vi "projekt2.vi"() -> ()   [LabVIEW 2020]
uses:
  6dc693d6-3625-4d42-a112-a50989b43f3c.vi
panel:
  in  "Precyzja":sgl min=0 max=6 step=1 format="%#_1g"
  out "Wynikk":string
  in  "Tryb":bool
  out "Wyniki":dbl(graph)
  out "Nieprawid³owa \nkonwersja":bool
  in  "Skala temperatury":bool
  in  "?":bool
  in  "stop":bool
  in  "Model [0-1]":u8 max=1 step=1
  in  "Rezystancja [DBL]":dbl format="%#.6g"
  in  "Jednostka [0-2]":u8 max=2 step=1
  # "Rezystancja"
  # "Temperatura"
  # "Czujnik"
  # "PT100"
  # "KTY81-210"
  # "Celcjusza"
  # "Fahrenheita"
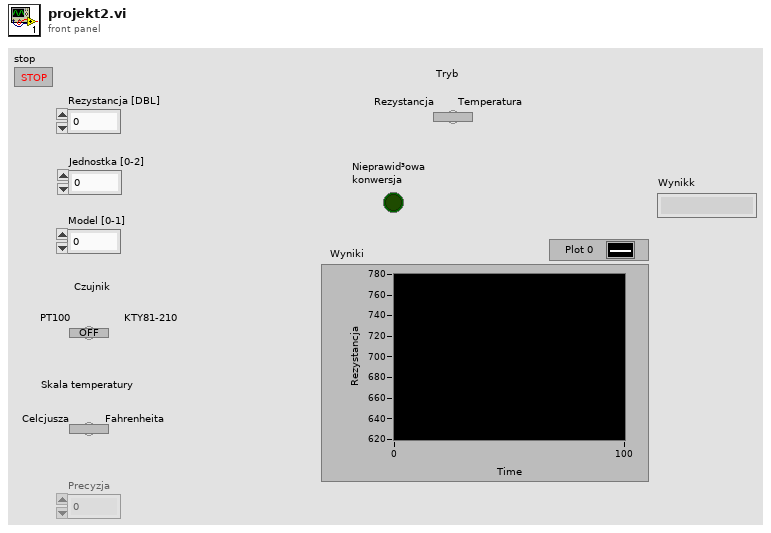
[diagram p1: front panel]
types:
  T1 = enum8{"Enabled", "Disabled", "Disabled and Grayed Out"}
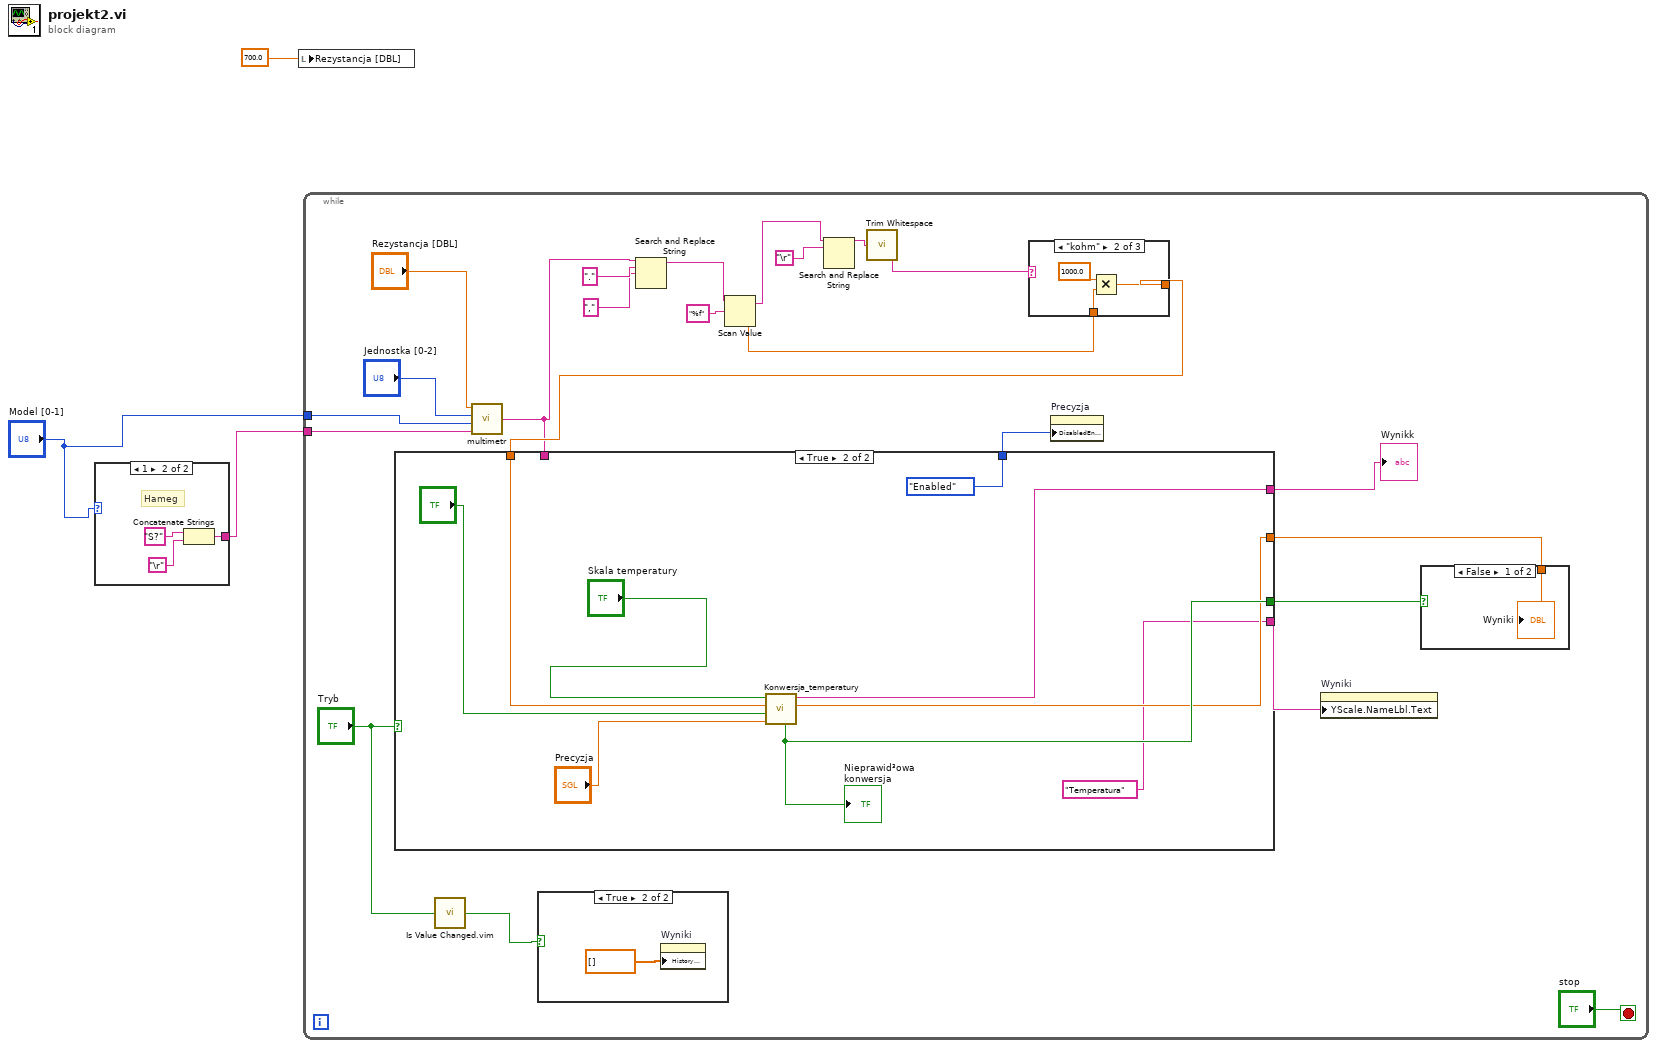
[diagram p0: block diagram]
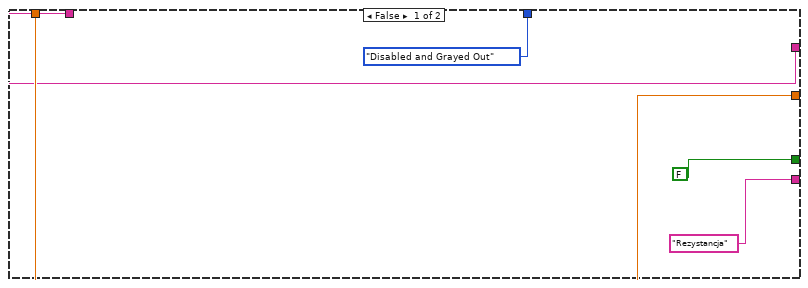
[diagram p4: hidden frame]
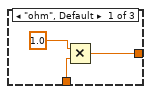
[diagram p5: hidden frame]
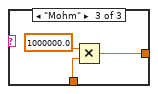
[diagram p6: hidden frame]
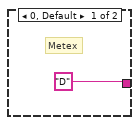
[diagram p7: hidden frame]
diagram:
  n1 = case shown="1" "Model [0-1]" {
    tunnel: ["D" w5] -> w2
    frame 0, Default {
      # "Metex"
    }
    frame 1 {
      # "Hameg"
      n2 = Concatenate Strings("S?", "\r") -> (w5:string)
    }
  }
  n3 = local write "Rezystancja [DBL]"(700.0 ("Rezystancja [DBL]")) -> ()
  n4 = while {
    tunnel: "Model [0-1]" -> [w30]
    tunnel: w2 -> [w29]
    stop <- "stop" stop-if-true
    n5 = call "Is Value Changed.vim"("value"="Tryb") -> ("changed or first call?"=w9:bool)
    n6 = call "multimetr.vi"("Zapytanie"=w29, "Model [0-1]"=w30, "Jednostka [0-2]"="Jednostka [0-2]", "Rezystancja [DBL]"="Rezystancja [DBL]") -> ("Ramka"=w12:string)
    n7 = case shown="True" w9 {
      frame False {
      }
      frame True {
        n8 = property on="Wyniki" class="WFChart (strict)"("History Data"=dbl[] []) -> ()  [unwired: 2 in, 2 out]
      }
    }
    n9 = Search and Replace String(input string=w12, search string=".", replace string=",") -> (result string=w26:string)  [unwired: 5 in, 3 out]
    n10 = Scan Value(string=w26, format string="%f") -> (output string=w21:string, value=w22:dbl)  [unwired: 1 in]
    n11 = Search and Replace String(input string=w21, search string="\r") -> (result string=w18:string)  [unwired: 6 in, 3 out]
    n12 = call <vilib>:"Trim Whitespace.vi"("string"=w18) -> ("trimmed string"=w14:string)  [unwired: 1 in]
    n13 = case shown="\"kohm\"" w14 {
      tunnel: w22 -> [w48 w51 w54]
      tunnel: [w47 w50 w53] -> w17
      frame "ohm", Default {
        n14 = Multiply(x=1.0, y=w48) -> (x*y=w47:dbl)
      }
      frame "kohm" {
        n15 = Multiply(x=1000.0, y=w51) -> (x*y=w50:dbl)
      }
      frame "Mohm" {
        n16 = Multiply(x=1000000.0, y=w54) -> (x*y=w53:dbl)
      }
    }
    n17 = case shown="True" "Tryb" {
      tunnel: w17 -> [w36 w45]
      tunnel: [FALSE w42] -> w16
      tunnel: [w36 w41] -> w15
      tunnel: [w35 w43] -> w13
      tunnel: w12 -> [w35 _]
      tunnel: ["Rezystancja" "Temperatura"] -> w11
      tunnel: [T1."Disabled and Grayed Out" ("Disabled") T1."Enabled" ("Disabled")] -> w8
      frame False {
      }
      frame True {
        n18 = call "Konwersja_temperatury.vi"("Precyzja"="Precyzja", 9:"?", "Rezystancja"=w45, "Skala temperatury"="Skala temperatury") -> ("Numeric"=w41:dbl, "String"=w43:string, "Nieprawid³owa \nkonwersja"=w42:bool)  [unwired: 5 in]
        "Nieprawid³owa \nkonwersja" <- w42
      }
    }
    "Wynikk" <- w13
    n19 = property on="Precyzja" class="DigNum (strict)"("DisabledEnum"=w8) -> ()  [unwired: 2 in, 2 out]
    n20 = property on="Wyniki" class="WFChart (strict)"("YScale.NameLbl.Text"=w11) -> ()  [unwired: 2 in, 2 out]
    n21 = case shown="False" w16 {
      tunnel: w15 -> [w32 _]
      frame False {
        "Wyniki" <- w32
      }
      frame True {
      }
    }
  }
